vi "single_color_2D_AFM_synched.vi"() -> ()   [LabVIEW 2017]
uses:
  <vilib>/DAQmx/write.llb/DAQmx Write (Analog DBL 1Chan 1Samp).vi
  <vilib>/DAQmx/write.llb/DAQmx Write (Analog 2D DBL NChan NSamp).vi
  <vilib>/DAQmx/write.llb/DAQmx Write (Analog 1D DBL NChan 1Samp).vi
  <vilib>/DAQmx/create/channels.llb/DAQmx Create Channel (AO-Voltage-Basic).vi
  <vilib>/DAQmx/miscellaneous.llb/DAQmx Fill In Error Info.vi
  <vilib>/DAQmx/configure/timing.llb/DAQmx Timing (Sample Clock).vi
  <vilib>/DAQmx/configure/trigger.llb/DAQmx Start Trigger (Digital Edge).vi
  <resource>/objmgr/daqmx.rc
panel:
  out "Focal Distance (um)":dbl
  out "Diopter":dbl
  in  "ETL3 (v)":dbl(slide)=4.76 caption="[4.76V allows light passing through unaltered]" min=-10.0 max=10.0 step=0.01 scale=-10.0..10.0
  in  "Y multiplier":dbl=1.0
  in  "X multiplier":dbl=-1.0
  in  "Y (v)":dbl(slide) min=-10.0 max=10.0 step=0.01 scale=-10.0..10.0
  in  "X (v)":dbl(slide) min=-10.0 max=10.0 step=0.01 scale=-10.0..10.0
  in  "Combined Movement (v)\nEquation: X * X Multiplier + Y * Y Multiplier":dbl(slide) min=-10.0 max=10.0 step=0.01 scale=-10.0..10.0
  out "Expected AFM Frequency (HZ)":dbl
  in  "Listbox":i32(listbox)=1
  in  "Laser 1 (0-10v)":dbl=3.0
  in  "OFF Time(ms)":dbl=100.0
  in  "ON Time(ms)":dbl=300.0
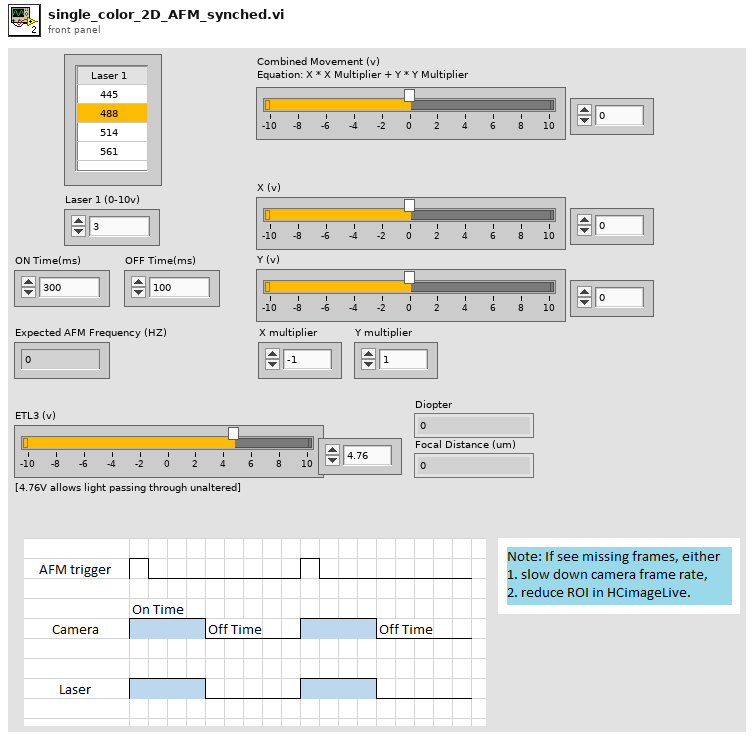
[diagram p1: front panel]
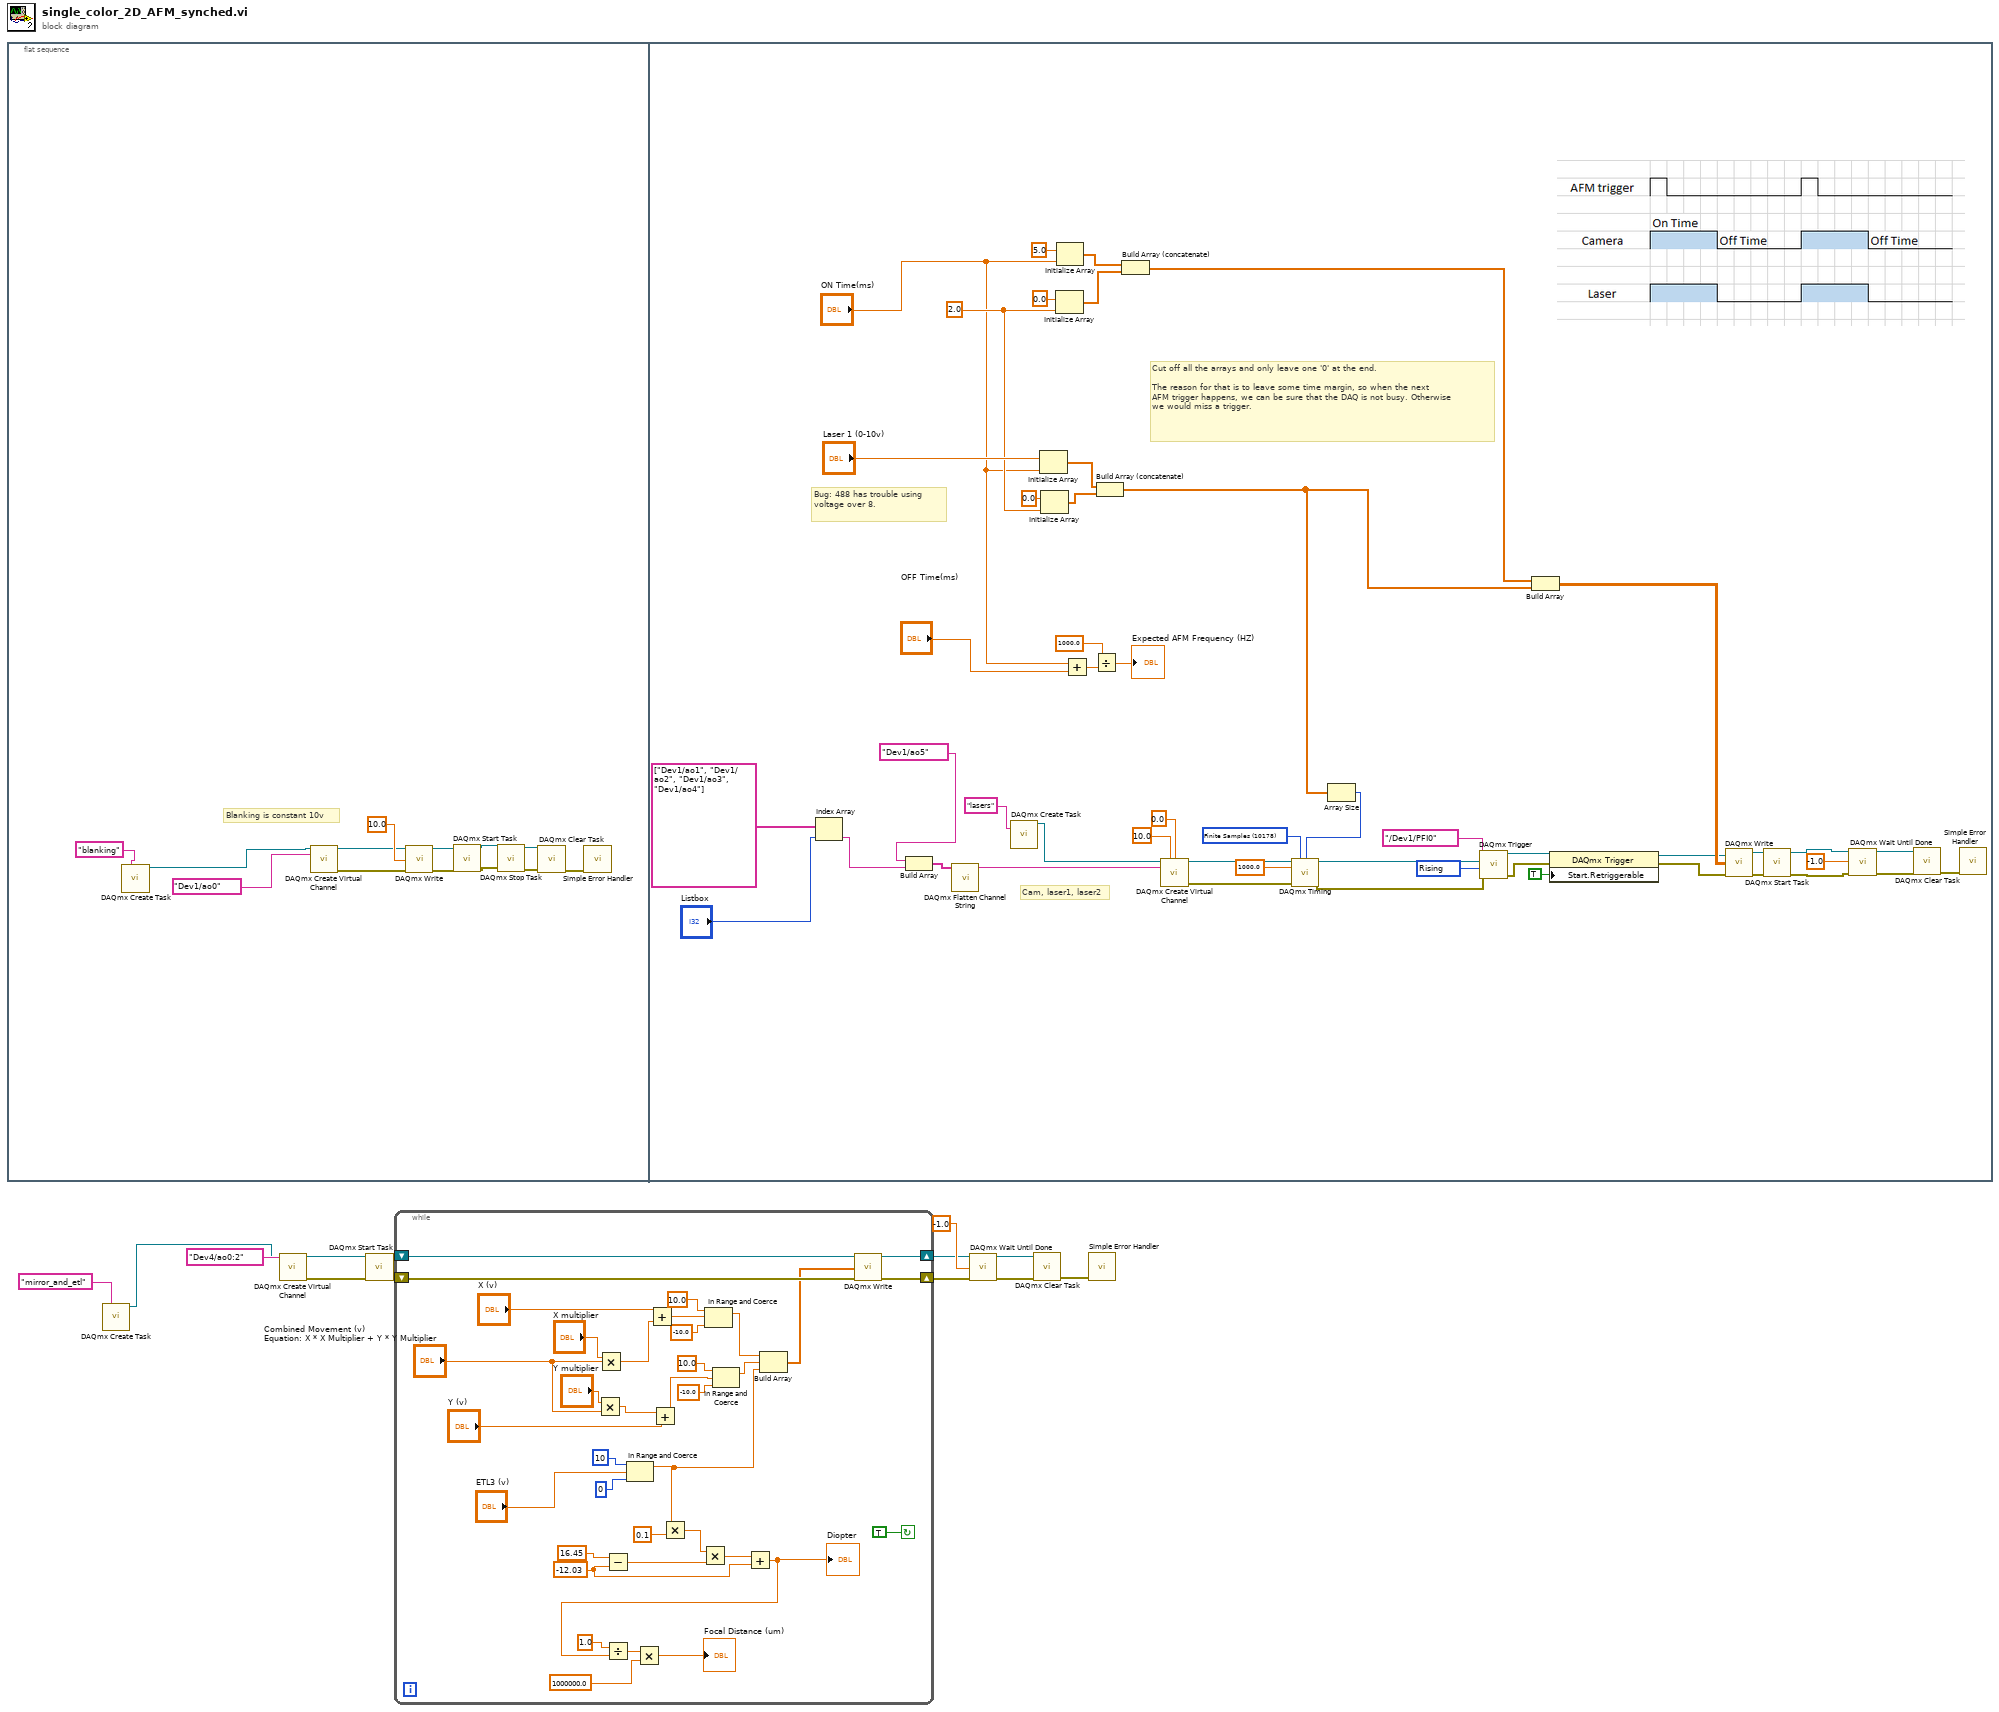
[diagram p0: block diagram]
diagram:
  n1 = flat-sequence {
    frame #0 {
      # "Blanking is constant 10v"
      n2 = call <vilib>:"DAQmx Create Task.vi"("new task name"="blanking" ("name to assign")) -> ("task out"=w16:refnum<k21>)  [unwired: 13 in, 1 out]
      n3 = call-poly <vilib>:"DAQmx Create Virtual Channel.vi"("task in"=w16, "physical channels"=tag "Dev1/ao0") -> ("task out"=w24:refnum<k21>, "error out"=w23:errorcluster)  [unwired: 12 in]
      n4 = call-poly <vilib>:"DAQmx Write.vi"("task/channels in"=w24, "data"=10.0, "error in"=w23) -> ("task out"=w22:refnum<k21>, "error out"=w21:errorcluster)  [unwired: 10 in, 1 out]
      n5 = call <vilib>:"DAQmx Start Task.vi"("task/channels in"=w22, "error in"=w21) -> ("task out"=w15:refnum<k21>, "error out"=w14:errorcluster)  [unwired: 12 in]
      n6 = call <vilib>:"DAQmx Stop Task.vi"("task/channels in"=w15, "error in"=w14) -> ("task out"=w20:refnum<k21>, "error out"=w19:errorcluster)  [unwired: 12 in]
      n7 = call <vilib>:"DAQmx Clear Task.vi"("task in"=w20, "error in"=w19) -> ("error out"=w26:errorcluster)  [unwired: 13 in]
      n8 = call <vilib>:"Simple Error Handler.vi"("error in (no error)"=w26) -> ()  [unwired: 4 in, 5 out]
    }
    frame #1 {
      w32 = 2.0
      w41 = 10280 items=["Rising"=10280, "Falling"=10171] ("edge")
      w37 = 10178 items=["Finite Samples"=10178, "Continuous Samples"=10123, "Hardware Timed Single Point"=12522] ("sample mode")
      # "Bug: 488 has trouble using voltage over 8."
      # "Cut off all the arrays and only leave one '0' at the end.\n\nThe reason for that is to leave some time margin, so when the next \nAFM trigger happens, we can be sure that the DAQ is not busy. Otherwise\nwe would miss a trigger."
      # "Cam, laser1, laser2"
      n9 = Index Array(array=tag[] ["Dev1/ao1", "Dev1/ao2", "Dev1/ao3", "Dev1/ao4"], index="Listbox") -> (element=w70:tag)
      n10 = Build Array(tag "Dev1/ao5" ("physical channels"), w70) -> (w71:tag[])
      n11 = call <vilib>:"DAQmx Flatten Channel String.vi"("names in"=w71) -> ("names out"=w73:string)  [unwired: 13 in, 1 out]
      n12 = call <vilib>:"DAQmx Create Task.vi"("new task name"="lasers" ("name to assign")) -> ("task out"=w75:refnum<k21>)  [unwired: 13 in, 1 out]
      n13 = Initialize Array("Laser 1 (0-10v)", "ON Time(ms)") -> (w49:dbl[])
      n14 = Initialize Array(0.0 ("element"), w32) -> (w50:dbl[])
      n15 = Initialize Array(0.0 ("element"), w32) -> (w31:dbl[])
      n16 = Initialize Array(5.0 ("element"), "ON Time(ms)") -> (w48:dbl[])
      n17 = Add(x="ON Time(ms)", y="OFF Time(ms)") -> (x+y=w66:dbl)
      n18 = Divide(x=1000.0, y=w66) -> (x/y=→"Expected AFM Frequency (HZ)":dbl)
      n19 = Build Array (concatenate)(w49, w50) -> (w27:dbl[])
      n20 = Build Array (concatenate)(w48, w31) -> (w30:dbl[])
      n21 = call-poly <vilib>:"DAQmx Create Virtual Channel.vi"("task in"=w75, "maximum value"=10.0, "minimum value"=0.0, "physical channels"=w73) -> ("task out"=w58:refnum<k21>, "error out"=w59:errorcluster)  [unwired: 10 in]
      n22 = Array Size(array=w27) -> (size(s)=w74:i32)
      n23 = call-poly <vilib>:"DAQmx Timing.vi"("task/channels in"=w58, "sample mode"=w37, "samples per channel"=w74, "rate"=1000.0, "error in"=w59) -> ("task out"=w60:refnum<k21>, "error out"=w61:errorcluster)  [unwired: 9 in]
      n24 = call-poly <vilib>:"DAQmx Trigger.vi"("task/channels in"=w60, "source"=tag "/Dev1/PFI0", "edge"=w41, "error in"=w61) -> ("task out"=w62:refnum<k21>, "error out"=w65:errorcluster)  [unwired: 10 in]
      n25 = Build Array(w30, w27) -> (w67:dbl[][])
      n26 = property class="DAQmx Trigger"(reference=w62, error in=w65, "Start.Retriggerable"=TRUE) -> (reference out=w63:refnum<k21>, error out=w64:errorcluster)
      n27 = call-poly <vilib>:"DAQmx Write.vi"("task/channels in"=w63, "data"=w67, "error in"=w64) -> ("task out"=w56:refnum<k21>, "error out"=w57:errorcluster)  [unwired: 10 in, 1 out]
      n28 = call <vilib>:"DAQmx Start Task.vi"("task/channels in"=w56, "error in"=w57) -> ("task out"=w55:refnum<k21>, "error out"=w54:errorcluster)  [unwired: 12 in]
      n29 = call <vilib>:"DAQmx Wait Until Done.vi"("task/channels in"=w55, "timeout (sec)"=-1.0, "error in"=w54) -> ("task out"=w52:refnum<k21>, "error out"=w53:errorcluster)  [unwired: 11 in]
      n30 = call <vilib>:"DAQmx Clear Task.vi"("task in"=w52, "error in"=w53) -> ("error out"=w51:errorcluster)  [unwired: 13 in]
      n31 = call <vilib>:"Simple Error Handler.vi"("error in (no error)"=w51) -> ()  [unwired: 4 in, 5 out]
    }
  }
  n32 = call <vilib>:"DAQmx Create Task.vi"("new task name"="mirror_and_etl" ("name to assign")) -> ("task out"=w1:refnum<k21>)  [unwired: 13 in, 1 out]
  n33 = call-poly <vilib>:"DAQmx Create Virtual Channel.vi"("task in"=w1, "physical channels"=tag "Dev4/ao0:2") -> ("task out"=w6:refnum<k21>, "error out"=w5:errorcluster)  [unwired: 12 in]
  n34 = call <vilib>:"DAQmx Start Task.vi"("task/channels in"=w6, "error in"=w5) -> ("task out"=w8:refnum<k21>, "error out"=w7:errorcluster)  [unwired: 12 in]
  n35 = while {
    shift-right: [w109] -> w3
    shift-left: w8 -> [w111]
    shift-right: [w108] -> w4
    shift-left: w7 -> [w110]
    stop <- TRUE continue-if-true
    w85 = -12.03 ("x")
    n36 = Multiply(x="Y multiplier", y="Combined Movement (v)\nEquation: X * X Multiplier + Y * Y Multiplier") -> (x*y=w96:dbl)
    n37 = Multiply(x="X multiplier", y="Combined Movement (v)\nEquation: X * X Multiplier + Y * Y Multiplier") -> (x*y=w105:dbl)
    n38 = Subtract(x=16.45 ("y"), y=w85) -> (x-y=w87:dbl)
    n39 = In Range and Coerce(upper limit=10, x="ETL3 (v)", lower limit=0) -> (coerced(x)=w84:dbl)  [unwired: 1 out]
    n40 = Add(x="X (v)", y=w105) -> (x+y=w104:dbl)
    n41 = Add(x=w96, y="Y (v)") -> (x+y=w98:dbl)
    n42 = Multiply(x=w84, y=0.1) -> (x*y=w88:dbl)
    n43 = Multiply(x=w88, y=w87) -> (x*y=w86:dbl)
    n44 = In Range and Coerce(upper limit=10.0, x=w104, lower limit=-10.0) -> (coerced(x)=w101:dbl)  [unwired: 1 out]
    n45 = In Range and Coerce(upper limit=10.0, x=w98, lower limit=-10.0) -> (coerced(x)=w97:dbl)  [unwired: 1 out]
    n46 = Add(x=w86, y=w85) -> (x+y=w79:dbl)
    "Diopter" <- w79
    n47 = Divide(x=1.0, y=w79) -> (x/y=w94:dbl)
    n48 = Multiply(x=w94, y=1000000.0) -> (x*y=→"Focal Distance (um)":dbl)
    n49 = Build Array(w101, w97, w84) -> (w107:dbl[])
    n50 = call-poly <vilib>:"DAQmx Write.vi"("task/channels in"=w111, "data"=w107, "error in"=w110) -> ("task out"=w109:refnum<k21>, "error out"=w108:errorcluster)  [unwired: 10 in, 1 out]
  }
  n51 = call <vilib>:"DAQmx Wait Until Done.vi"("task/channels in"=w3, "timeout (sec)"=-1.0, "error in"=w4) -> ("task out"=w12:refnum<k21>, "error out"=w11:errorcluster)  [unwired: 11 in]
  n52 = call <vilib>:"DAQmx Clear Task.vi"("task in"=w12, "error in"=w11) -> ("error out"=w13:errorcluster)  [unwired: 13 in]
  n53 = call <vilib>:"Simple Error Handler.vi"("error in (no error)"=w13) -> ()  [unwired: 4 in, 5 out]
